vi "Clear-reference.vi"(8 "error in (no error)":errorcluster, 10 "Object reference":T1) -> (0 "error out":errorcluster, 3 "SM1000-control out":refnum<class "HC-SM1000.lvclass">)   [LabVIEW 2013, in "HardwareCharacterization.lvlib" / "HC-SM1000.lvclass"]
uses:
  HC-SM1000.lvclass
  Object-reference.ctl
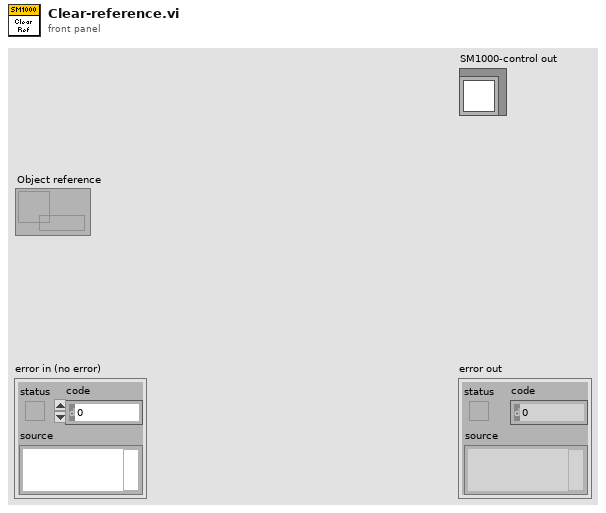
[diagram p1: front panel]
types:
  T1 = typedef "HardwareCharacterization.lvlib/HC-SM1000.lvclass/Object-reference.ctl" = refnum<data-value>
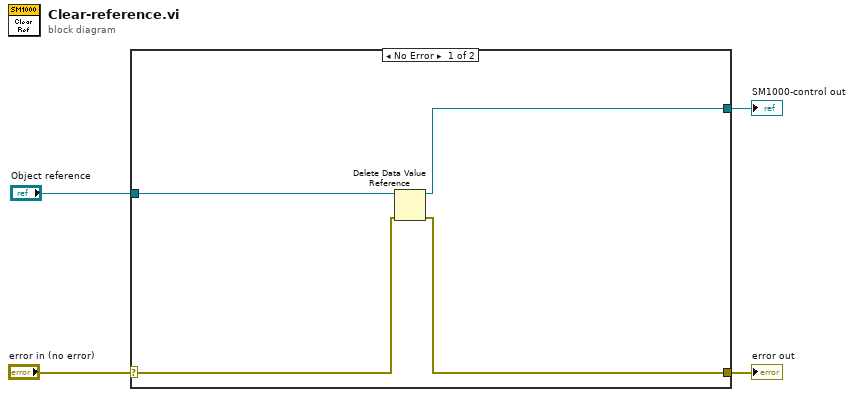
[diagram p0: block diagram]
diagram:
  n1 = case shown="No Error" "error in (no error)" {
    selector: "error in (no error)" -> [w8 w9]
    tunnel: [w7 w9] -> w3
    tunnel: [w5 _] -> w2
    tunnel: "Object reference" -> [w6 _]
    frame No Error {
      n2 = Delete Data Value Reference(data value reference=w6, error in=w8) -> (data value=w5:refnum<class "HC-SM1000.lvclass">, error out=w7:errorcluster)
    }
    frame Error {
    }
  }
  "error out" <- w3
  "SM1000-control out" <- w2
